vi "v0.2_lee_RPM_serial.vi"(8 "error in (no error)":errorcluster, 11 "VISA COM IN":refnum<visa-resource-name>) -> (0 "error out":errorcluster, 2 "RPM":dbl, 3 "VISA COM OUT":refnum<visa-resource-name>)   [LabVIEW 2011]
doc: "<B>PTO Salida de tren de pulsos</B>\n\nCambiar la frecuencia de salida. Un valor de cero detiene el motor. Existe un valor máximo luego del cual el servomotor se detiene, este valor depende de los paràmetros del driver.\n<B>Frecuencia </B> Valor en hertzios del tren de pulsos a la salida del microcontrolador mbed."
panel:
  # "Leer el velocidad  del encoder en RPM's"
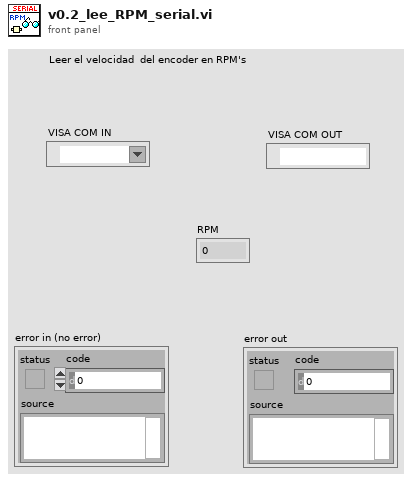
[diagram p1: front panel]
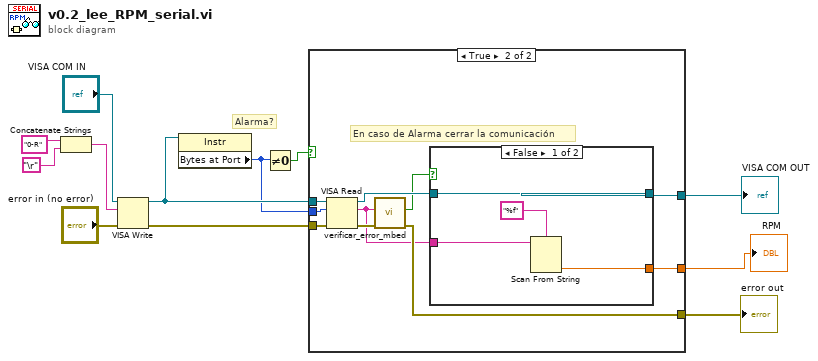
[diagram p0: block diagram]
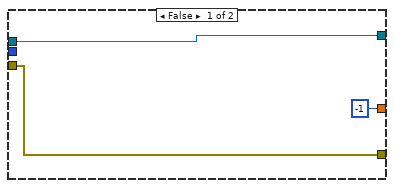
[diagram p2: hidden frame]
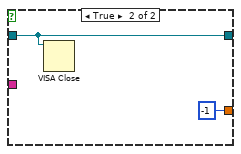
[diagram p3: hidden frame]
diagram:
  # "Alarma?"
  n1 = Concatenate Strings("0-R" ("string"), "\r") -> (w11:string)
  n2 = VISA Write(VISA resource name="VISA COM IN", write buffer=w11, error in (no error)="error in (no error)") -> (VISA resource name out=w6:refnum<visa-resource-name>, error out=w8:errorcluster)  [unwired: 1 out]
  n3 = property class="Instr"(reference=w6) -> ("Bytes at Port"=w4:u32)  [unwired: 1 in, 2 out]
  n4 = Not Equal To 0?(x=w4) -> (x != 0?=w5:bool)
  n5 = case shown="True" w5 {
    tunnel: w6 -> [w15 w23]
    tunnel: w8 -> [w14 w22]
    tunnel: w4 -> [_ w20]
    tunnel: [w15 w19] -> w3
    tunnel: [w14 w18] -> w2
    tunnel: [-1 w16] -> w1
    frame False {
    }
    frame True {
      # "En caso de Alarma cerrar la comunicación"
      n6 = VISA Read(VISA resource name=w23, byte count=w20, error in (no error)=w22) -> (VISA resource name out=w24:refnum<visa-resource-name>, read buffer=w17:string, error out=w25:errorcluster)  [unwired: 1 out]
      n7 = call "verificar_error_mbed.vi"("error in (no error)"=w25, "desde_mbed"=w17) -> ("error out"=w18:errorcluster, "error?"=w21:bool)  [unwired: 8 in]
      n8 = case shown="False" w21 {
        tunnel: w24 -> [w29 w31]
        tunnel: [w29 w31] -> w19
        tunnel: w17 -> [w28 _]
        tunnel: [w26 -1] -> w16
        frame False {
          n9 = Scan From String(format string="%f", input string=w28) -> (output 1=w26:dbl)  [unwired: 3 in, 3 out]
        }
        frame True {
          n10 = VISA Close(VISA resource name=w31) -> ()  [unwired: 1 in, 1 out]
        }
      }
    }
  }
  "VISA COM OUT" <- w3
  "error out" <- w2
  "RPM" <- w1
